vi "TCPIP.Server v2.vi"() -> ()   [LabVIEW 2019]
panel:
  in  "port":u16=50009
  in  "Log_file":path=path "D:/DNN_data/20170731_testrun.txt"
  out "Client Connected":bool=TRUE
  out "Command (from Python)":string="hello(world)\r\n"
  out "Return Value String (for Python)":string="Hello world"
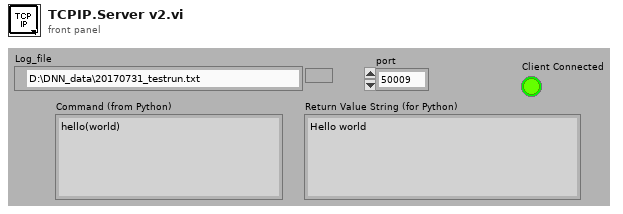
[diagram p1: front panel]
types:
  T1 = enum16{"Standard", "Buffered", "CRLF", "Immediate"}
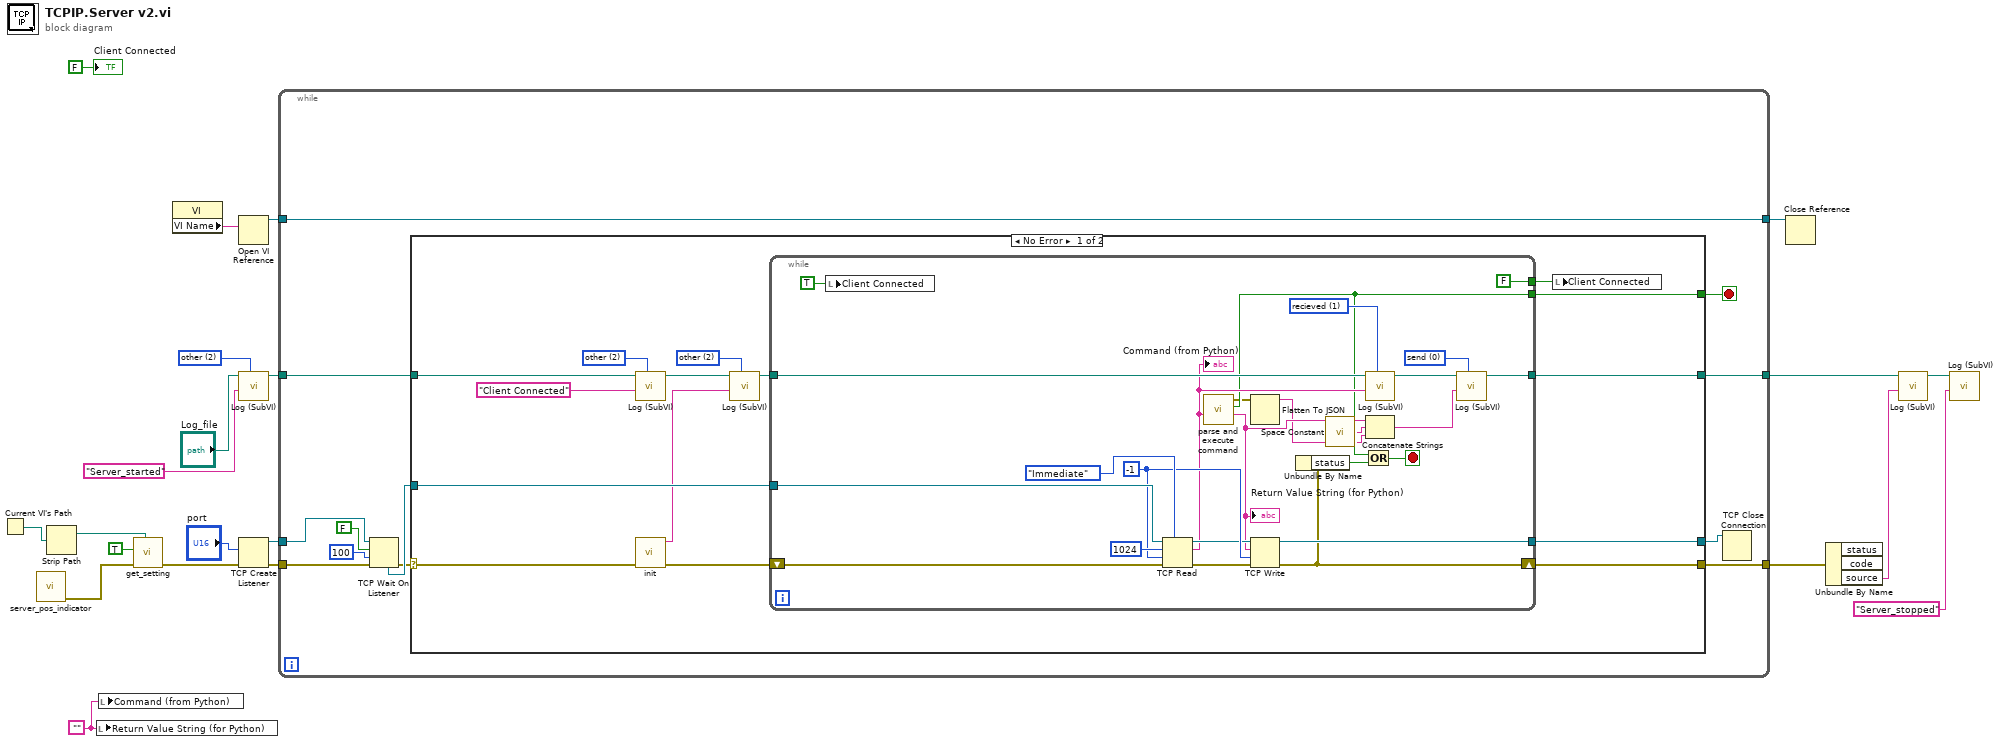
[diagram p0: block diagram]
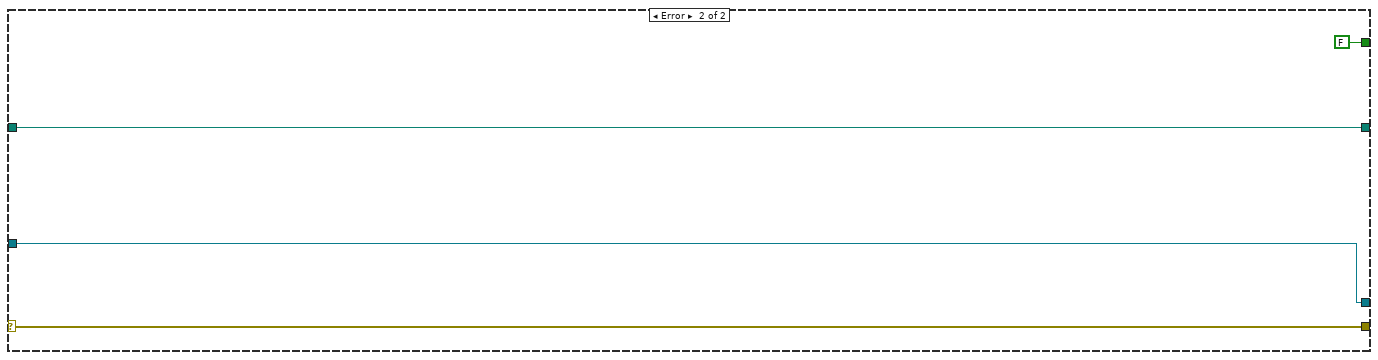
[diagram p2: hidden frame]
diagram:
  w12 = u16 2 items=["send", "recieved", "other"] ("Msgtype")
  w18 = ""
  n1 = Current VI's Path() -> (path=w2:path)
  n2 = call "server_pos_indicator.vi"() -> ("error out"=w3:errorcluster)  [unwired: 11 in]
  n3 = Strip Path(path=w2) -> (stripped path=w1:path)  [unwired: 1 out]
  n4 = local write "Return Value String (for Python)"(w18) -> ()
  n5 = local write "Command (from Python)"(w18) -> ()
  n6 = call "get_setting.vi"("settings path"=w1, "error in (no error)"=w3, "FirstRun"=TRUE) -> ("error out"=w5:errorcluster)  [unwired: 4 in, 4 out]
  n7 = property class="VI"() -> ("VI Name"=w21:string)  [unwired: 2 in, 2 out]
  n8 = Open VI Reference(vi path=w21) -> (vi reference=w20:refnum<vi>)  [unwired: 5 in, 1 out]
  n9 = call "Log (SubVI).vi"("Msgtype"=w12, "String"="Server_started", "file path (use dialog)"="Log_file") -> ("path"=w14:path)  [unwired: 8 in]
  n10 = TCP Create Listener(8:w5, 10:"port") -> (0:w22:errorcluster, 3:w15:refnum<k5>)  [unwired: 3 in, 1 out]
  n11 = while {
    tunnel: w20 -> [w29]
    tunnel: [w29] -> w19
    tunnel: w22 -> [w34]
    tunnel: w15 -> [w27]
    tunnel: w14 -> [w26]
    tunnel: [w25] -> w10
    tunnel: [w24] -> w9
    stop <- w23 stop-if-true
    n12 = TCP Wait On Listener(8:w34, 9:100 ("timeout ms (wait forever: -1)"), 10:FALSE ("resolve remote address (T)"), 11:w27) -> (0:w28:errorcluster, 4:w32:refnum<k5>)  [unwired: 3 out]
    n13 = case shown="No Error" w28 {
      selector: w28 -> [w43 w76]
      tunnel: w32 -> [w49 w78]
      tunnel: [w48 w78] -> w31
      tunnel: w26 -> [w38 w77]
      tunnel: [w46 w77] -> w25
      tunnel: [w45 w76] -> w24
      tunnel: [w44 FALSE ("exit")] -> w23
      frame No Error {
        w35 = u16 2 items=["send", "recieved", "other"] ("Msgtype")
        w40 = u16 2 items=["send", "recieved", "other"] ("Msgtype")
        n14 = call "Log (SubVI).vi"("Msgtype"=w35, "String"="Client Connected", "file path (use dialog)"=w38) -> ("path"=w37:path)  [unwired: 8 in]
        n15 = call "init.vi"("error in (no error)"=w43) -> ("error out"=w42:errorcluster, "Output"=w39:string)  [unwired: 9 in]
        n16 = call "Log (SubVI).vi"("Msgtype"=w40, "String"=w39, "file path (use dialog)"=w37) -> ("path"=w41:path)  [unwired: 8 in]
        n17 = while {
          tunnel: [FALSE ("Connected")] -> w47
          shift-left: w42 -> [w50]
          shift-right: [w70] -> w45
          tunnel: [w71] -> w48
          tunnel: w49 -> [w72]
          tunnel: w41 -> [w65]
          tunnel: [w61] -> w46
          tunnel: [w56] -> w44
          stop <- w57 stop-if-true
          w62 = u16 0 items=["send", "recieved", "other"] ("Msgtype")
          w63 = u16 1 items=["send", "recieved", "other"] ("Msgtype")
          w67 = -1 ("timeout ms (25000)")
          n18 = local write "Client Connected"(TRUE ("Connected")) -> ()
          n19 = TCP Read(connection ID=w72, bytes to read=1024, error in (no error)=w50, 7:T1."Immediate" ("mode (standard)"), 9:w67) -> (connection ID out=w66:refnum<k5>, data out=w60:string, error out=w51:errorcluster)
          "Command (from Python)" <- w60
          n20 = call "parse and execute command.vi"("Python Command"=w60) -> ("Python Return String"=w59:string, "exit"=w56:bool, "command error"=w53:errorcluster)  [unwired: 7 in]
          "Return Value String (for Python)" <- w59
          n21 = Flatten To JSON(anything=w53) -> (JSON string=w52:string)  [unwired: 2 in, 1 out]
          n22 = TCP Write(connection ID=w66, data in=w59, error in (no error)=w51, 9:w67) -> (connection ID out=w71:refnum<k5>, error out=w70:errorcluster)  [unwired: 1 out]
          n23 = Unbundle By Name(w70) -> ("status"=w58:bool)
          n24 = call <vilib>:"Space Constant.vi"() -> ("String"=w54:string)
          n25 = Or(x=w56, y=w58) -> (x .or. y?=w57:bool)
          n26 = call "Log (SubVI).vi"("Msgtype"=w63, "String"=w60, "file path (use dialog)"=w65) -> ("path"=w64:path)  [unwired: 8 in]
          n27 = Concatenate Strings(w59, w54, w52) -> (w55:string)
          n28 = call "Log (SubVI).vi"("Msgtype"=w62, "String"=w55, "file path (use dialog)"=w64) -> ("path"=w61:path)  [unwired: 8 in]
        }
        n29 = local write "Client Connected"(w47) -> ()
      }
      frame Error {
      }
    }
    n30 = TCP Close Connection(connection ID=w31) -> ()  [unwired: 2 in, 2 out]
  }
  n31 = Close Reference(reference=w19) -> ()  [unwired: 1 in, 1 out]
  n32 = Unbundle By Name(w9) -> ("source"=w8:string)  [unwired: 2 out]
  n33 = call "Log (SubVI).vi"("String"=w8, "file path (use dialog)"=w10) -> ("path"=w7:path)  [unwired: 9 in]
  n34 = call "Log (SubVI).vi"("String"="Server_stopped", "file path (use dialog)"=w7) -> ()  [unwired: 9 in, 1 out]
  "Client Connected" <- FALSE ("Connected")
